vi "Attocube_to_DSC.vi"(4 "boolean var":refnum<k21>[](array[refnum])=["ni.var.psp://housesoftheholy/Attocube 3DR/axis 1%3A Target GND", "ni.var.psp://housesoftheholy/Attocube 3DR/axis 1%3A Output", "ni.var.psp://housesoftheholy/Attocube 3DR/axis 1%3A Single Circle Mode", "ni.var.psp://housesoftheholy/Attocube 3DR/axis 1%3A moving", "ni.var.psp://housesoftheholy/Attocube 3DR/axis 1%3A stop detected", "ni.var.psp://housesoftheholy/Attocube 3DR/axis 1%3A sensor error", "ni.var.psp://housesoftheholy/Attocube 3DR/axis 1%3A sensor disconnected", "ni.var.psp://housesoftheholy/Attocube 3DR/axis 1%3A stop enable", "ni.var.psp://housesoftheholy/Attocube 3DR/axis 2%3A Target GND", "ni.var.psp://housesoftheholy/Attocube 3DR/axis 2%3A Output", "ni.var.psp://housesoftheholy/Attocube 3DR/axis 2%3A Single Circle Mode", "ni.var.psp://housesoftheholy/Attocube 3DR/axis 2%3A moving", "ni.var.psp://housesoftheholy/Attocube 3DR/axis 2%3A stop detected", "ni.var.psp://housesoftheholy/Attocube 3DR/axis 2%3A sensor error", "ni.var.psp://housesoftheholy/Attocube 3DR/axis 2%3A sensor disconnected", "ni.var.psp://housesoftheholy/Attocube 3DR/axis 2%3A stop enable"], 5 "boolean":bool[](array[boolean])=[FALSE, FALSE, TRUE, FALSE, FALSE, FALSE, FALSE, TRUE, FALSE, FALSE, FALSE, FALSE, FALSE, FALSE, FALSE, TRUE], 6 "dbl var":refnum<k21>[](array[refnum])=["ni.var.psp://housesoftheholy/Attocube 3DR/axis 1%3A Amplitude", "ni.var.psp://housesoftheholy/Attocube 3DR/axis 1%3A Capacitance", "ni.var.psp://housesoftheholy/Attocube 3DR/axis 1%3A current position", "ni.var.psp://housesoftheholy/Attocube 3DR/axis 1%3A DCLevel", "ni.var.psp://housesoftheholy/Attocube 3DR/axis 1%3A Frequency", "ni.var.psp://housesoftheholy/Attocube 3DR/axis 1%3A StepWidth", "ni.var.psp://housesoftheholy/Attocube 3DR/axis 1%3A control mode", "ni.var.psp://housesoftheholy/Attocube 3DR/axis 1%3A rot. count", "ni.var.psp://housesoftheholy/Attocube 3DR/axis 1%3A sp position", "ni.var.psp://housesoftheholy/Attocube 3DR/axis 1%3A sp rot count", "ni.var.psp://housesoftheholy/Attocube 3DR/axis 1%3A speed", "ni.var.psp://housesoftheholy/Attocube 3DR/axis 2%3A Amplitude", "ni.var.psp://housesoftheholy/Attocube 3DR/axis 2%3A Capacitance", "ni.var.psp://housesoftheholy/Attocube 3DR/axis 2%3A current position", "ni.var.psp://housesoftheholy/Attocube 3DR/axis 2%3A DCLevel", "ni.var.psp://housesoftheholy/Attocube 3DR/axis 2%3A Frequency", "ni.var.psp://housesoftheholy/Attocube 3DR/axis 2%3A StepWidth", "ni.var.psp://housesoftheholy/Attocube 3DR/axis 2%3A control mode", "ni.var.psp://housesoftheholy/Attocube 3DR/axis 2%3A rot. count", "ni.var.psp://housesoftheholy/Attocube 3DR/axis 2%3A sp position", "ni.var.psp://housesoftheholy/Attocube 3DR/axis 2%3A sp rot count", "ni.var.psp://housesoftheholy/Attocube 3DR/axis 2%3A speed"], 7 "dbl":dbl[](array[numeric])=[30.0, 2725.0, 0.0, 0.0, 1000.0, 41.0, 1.0, 0.0, 30.0, 0.0, 33.0, 30.0, 2473.0, 0.0, 0.0, 1000.0, 9.0, 1.0, 0.0, 30.0, 0.0, 7.0]) -> ()   [LabVIEW 2013]
panel:
  # "Attocube to DSC"
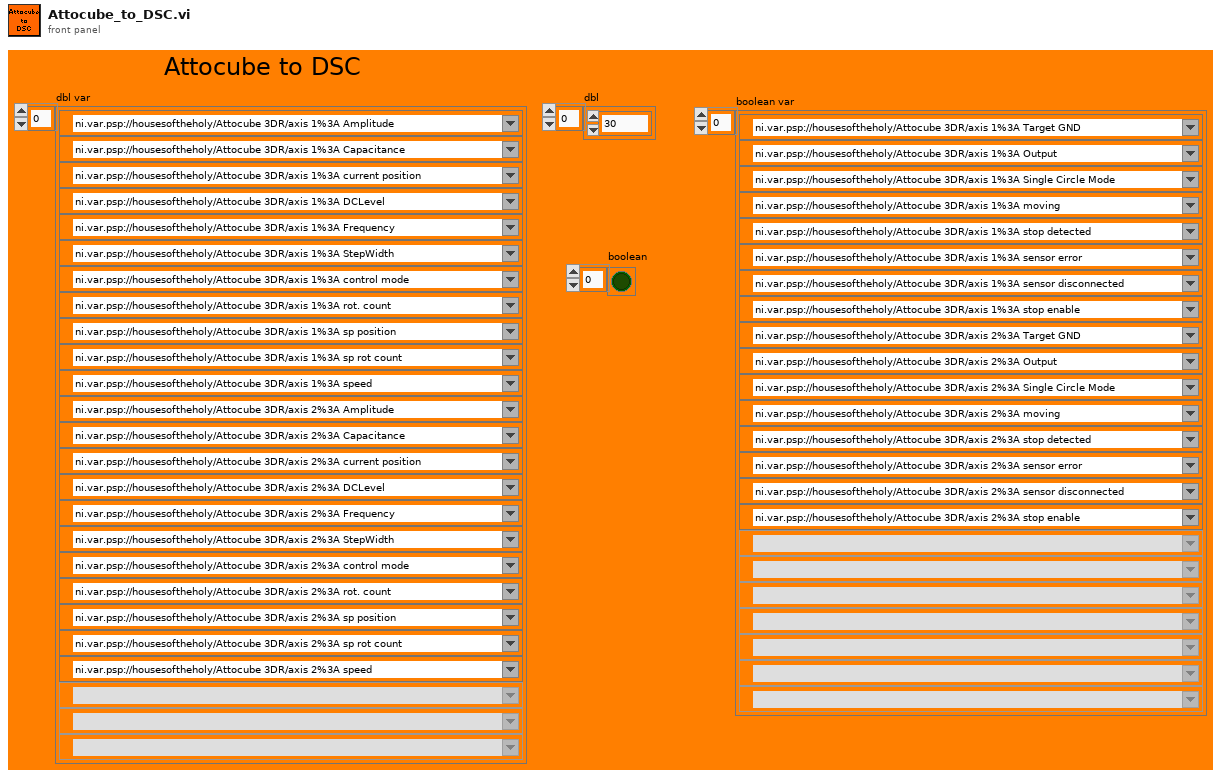
[diagram p1: front panel]
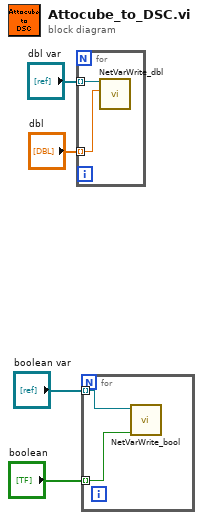
[diagram p0: block diagram]
diagram:
  n1 = for {
    tunnel: "dbl var" -> [w6] mode=indexing
    tunnel: "dbl" -> [w5] mode=indexing
    n2 = call "NetVarWrite_dbl.vi"("Numeric"=w5, "Refnum in"=w6) -> ()  [unwired: 10 in]
  }
  n3 = for {
    tunnel: "boolean" -> [w8] mode=indexing
    tunnel: "boolean var" -> [w7] mode=indexing
    n4 = call "NetVarWrite_bool.vi"("data in"=w8, "Refnum in"=w7) -> ()  [unwired: 10 in]
  }
